vi "Set Watchdog Interval.vi"(0 "VISA resource name":refnum<visa-resource-name>, 5 "Watchdog Interval (s)":dbl format="%#.6f", 11 "error in (no error)":errorcluster) -> (4 "VISA resource name out":refnum<visa-resource-name>, 15 "error out":errorcluster)   [LabVIEW 2012, in "NH Research Regenerative Test Series.lvlib"]
doc: "Specifies how often communications must take place before the Module shuts itself off. The communication required to reset the watchdog timer (and keep the Module working) depends on the Set Watchdog Robust command. If Robust is set to ON, only the Service Watchdog.vi will reset the timer. If robust is set to OFF (the default), any communication will reset the timer."
uses:
  <instrlib>/NH Research Regenerative Test Series/NH Research Regenerative Test Series.lvlib
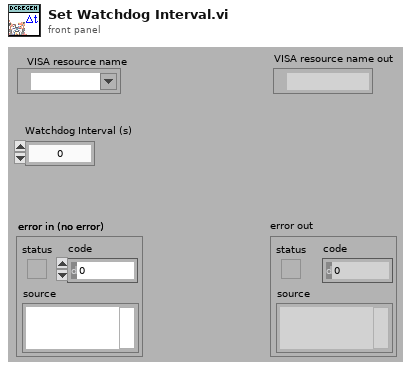
[diagram p1: front panel]
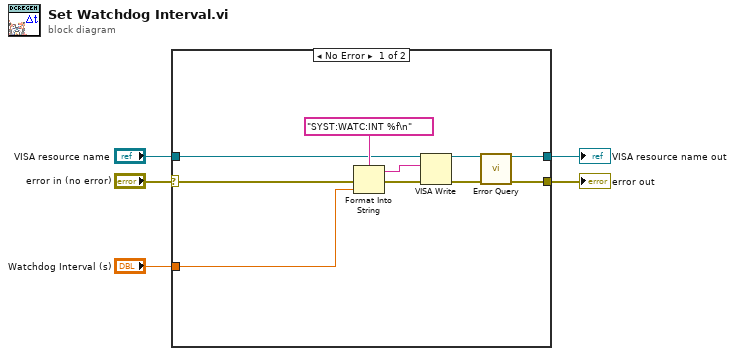
[diagram p0: block diagram]
diagram:
  n1 = case shown="No Error" "error in (no error)" {
    selector: "error in (no error)" -> [w10 w17]
    tunnel: "VISA resource name" -> [w9 w16]
    tunnel: [w15 w16] -> w4
    tunnel: [w14 w17] -> w3
    tunnel: "Watchdog Interval (s)" -> [w6 _]
    frame No Error {
      n2 = Format Into String(format string="SYST:WATC:INT %f\n" ("Command"), error in=w10, w6) -> (resulting string=w7:string, error out=w8:errorcluster)  [unwired: 1 in]
      n3 = VISA Write(VISA resource name=w9, write buffer=w7, error in (no error)=w8) -> (VISA resource name out=w13:refnum<visa-resource-name>, error out=w12:errorcluster)  [unwired: 1 out]
      n4 = call <instrlib>:"Error Query.vi"("VISA resource name"=w13, "error in (no error)"=w12) -> ("VISA resource name out"=w15:refnum<visa-resource-name>, "error out"=w14:errorcluster)  [unwired: 10 in, 2 out]
    }
    frame Error {
    }
  }
  "error out" <- w3
  "VISA resource name out" <- w4
